vi "TagContainer-New.vi"(8 "error in (no error)":errorcluster) -> (0 "error out":errorcluster, 3 "TagContainer":T1)   [LabVIEW 2017, in "TagContainer.lvlib"]
uses:
  TagContainer.lvlib
  Typedef/TagContainer.ctl
  Typedef/tagcontainer-data.ctl
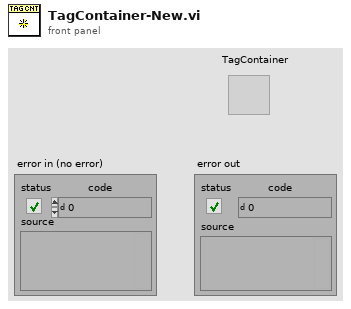
[diagram p1: front panel]
types:
  T1 = typedef "TagContainer.lvlib/TagContainer.ctl" = refnum<k1>
  T2 = typedef "TagContainer.lvlib/tagcontainer-data.ctl" = cluster{"tag-map":variant, "timestamp-map":variant, "namecacher-map":variant}
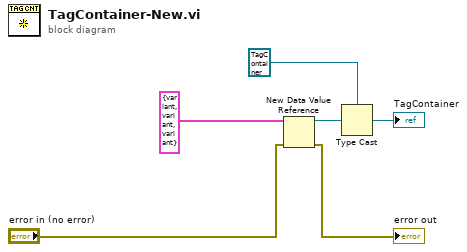
[diagram p0: block diagram]
diagram:
  n1 = New Data Value Reference(data value=T2 {"tag-map"=variant, "timestamp-map"=variant, "namecacher-map"=variant}, error in="error in (no error)") -> (data value reference=w4:refnum<data-value>, error out=→"error out":errorcluster)
  n2 = Type Cast(type=T1 refnum ("TagContainer"), x=w4) -> (*(type *) &x=→"TagContainer":T1)
